vi "AppleScript Main.vi"() -> ()   [LabVIEW 2016]
doc: "Main block for AppleScript.\nPut this in the autonomous vi. Do not place this inside of a loop."
panel:
  in  "auto mode":dbl
  # "AppleScript\nAutonomous Scripting Language for LabVIEW\nCreated by Cory Lynch\nFRC Team 2067"
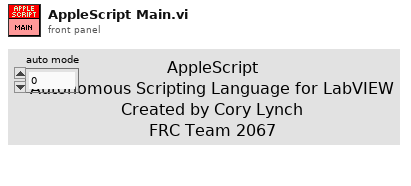
[diagram p1: front panel]
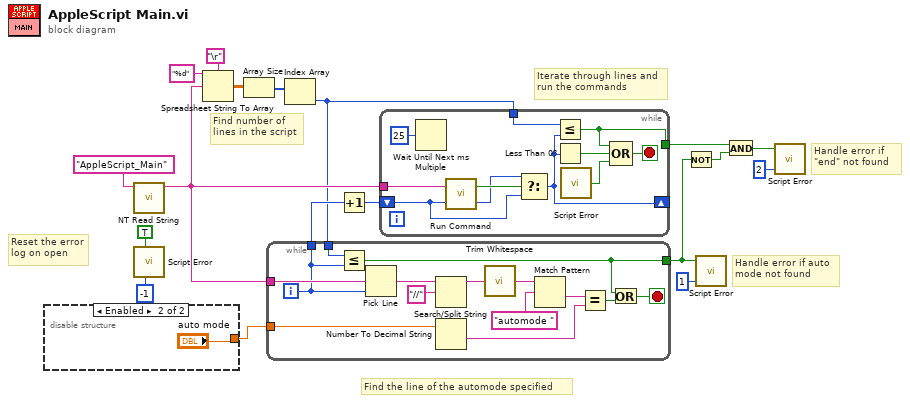
[diagram p0: block diagram]
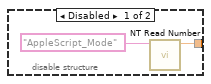
[diagram p2: hidden frame]
diagram:
  # "Find number of \nlines in the script"
  # "Handle error if\n\"end\" not found"
  # "Handle error if auto\nmode not found"
  # "Iterate through lines and\nrun the commands"
  # "Find the line of the automode specified"
  # "Reset the error\nlog on open"
  n1 = disable-structure shown="Enabled" {
    disable-tunnel: [w19 "auto mode"] -> w1
    frame Disabled {
      n2 = call <vilib>:"NT Read Number.vi"("Name"="AppleScript_Mode") -> ("Numeric"=w19:dbl)  [unwired: 9 in, 1 out]
    }
    frame Enabled {
    }
  }
  n3 = call <vilib>:"NT Read String.vi"("Name"="AppleScript_Main") -> ("String"=w12:string)  [unwired: 9 in, 1 out]
  n4 = call "Script Error.vi"("Reset Log"=TRUE, "Line Number"=-1) -> ()  [unwired: 3 in, 1 out]
  n5 = Spreadsheet String To Array(delimiter (Tab)="\r", format string="%d", spreadsheet string=w12) -> (array=w16:dbl[][])  [unwired: 1 in]
  n6 = Array Size(array=w16) -> (size(s)=w13:i32[])
  n7 = Index Array(array=w13) -> (element=w6:i32)  [unwired: 1 in]
  n8 = while {
    tunnel: w12 -> [w29]
    tunnel: [w25] -> w18
    tunnel: w6 -> [w26]
    tunnel: [w23] -> w5
    tunnel: w1 -> [w22]
    i -> [w25]
    stop <- w24 stop-if-true
    n9 = Less Or Equal?(x=w26, y=w25) -> (x <= y?=w23:bool)
    n10 = Pick Line(multi-line string=w29, line index=w25) -> (output string=w28:string)  [unwired: 1 in]
    n11 = Search/Split String(string=w28, search string/char (-)="//") -> (substring before match=w31:string)  [unwired: 1 in, 2 out]
    n12 = Number To Decimal String(number=w22) -> (decimal integer string=w33:string)  [unwired: 1 in]
    n13 = call <vilib>:"Trim Whitespace.vi"("string"=w31) -> ("trimmed string"=w30:string)  [unwired: 1 in]
    n14 = Match Pattern(string=w30, regular expression="automode ") -> (after substring=w34:string)  [unwired: 1 in, 3 out]
    n15 = Equal?(x=w34, y=w33) -> (x = y?=w27:bool)
    n16 = Or(x=w23, y=w27) -> (x .or. y?=w24:bool)
  }
  n17 = Increment(x=w18) -> (x+1=w3:i32)
  n18 = while {
    tunnel: w12 -> [w46]
    shift-right: [w43] -> _
    shift-left: w3 -> [w45]
    tunnel: w6 -> [w42]
    tunnel: [w41] -> w9
    stop <- w39 stop-if-true
    n19 = Wait Until Next ms Multiple(millisecond multiple=u32 25 ("milliseconds to wait")) -> ()  [unwired: 1 out]
    n20 = call "Run Command.vi"("Line Index In"=w45, "Script"=w46) -> ("Line Index Out"=w36:i32, "Done"=w44:bool)
    n21 = Select(t=w36, s=w44, f=w45) -> (s? t:f=w43:i32)
    n22 = Less Or Equal?(x=w42, y=w43) -> (x <= y?=w41:bool)
    n23 = Less Than 0?(x=w43) -> (x < 0?=w40:bool)
    n24 = call "Script Error.vi"() -> ("Error?"=w38:bool)  [unwired: 5 in]
    n25 = Compound Arithmetic op=OR(w41, w40, w38) -> (w39:bool)
  }
  n26 = Not(x=w5) -> (.not. x?=w8:bool)
  n27 = call "Script Error.vi"("Error?"=w5, "Error Code"=1) -> ()  [unwired: 3 in, 1 out]
  n28 = And(x=w9, y=w8) -> (x .and. y?=w7:bool)
  n29 = call "Script Error.vi"("Error?"=w7, "Error Code"=2) -> ()  [unwired: 3 in, 1 out]
